vi "计数器.vi"(7 "Reset":bool, 10 "次数":i32, 11 "UP?":bool) -> (3 "大于?":bool)   [LabVIEW 2017]
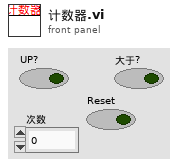
[diagram p1: front panel]
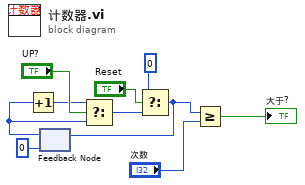
[diagram p0: block diagram]
diagram:
  n1 = feedback #1(0) -> (w7:i32)
  n2 = Increment(x=w7) -> (x+1=w6:i32)
  n3 = Select(t=w6, s="UP?", f=w7) -> (s? t:f=w4:i32)
  n4 = Select(t=0, s="Reset", f=w4) -> (s? t:f=w1:i32)
  n5 = feedback-in #1(w1) -> ()
  n6 = Greater Or Equal?(x=w1, y="次数") -> (x >= y?=→"大于?":bool)
